vi "STATUS_API.vi"(0 "modpath":path, 7 "Cmd":string, 11 "error in":errorcluster) -> (4 "ImmedReplyString":string, 15 "error out":errorcluster)   [LabVIEW 2016]
uses:
  DBSHAND/private/vis/DatabaseHand_Element_Set(string).vi
  DBSHAND/private/vis/DatabaseHand_Element_Set(bool).vi
panel:
  in  "Status server name":string="STATUS_Main.vi"
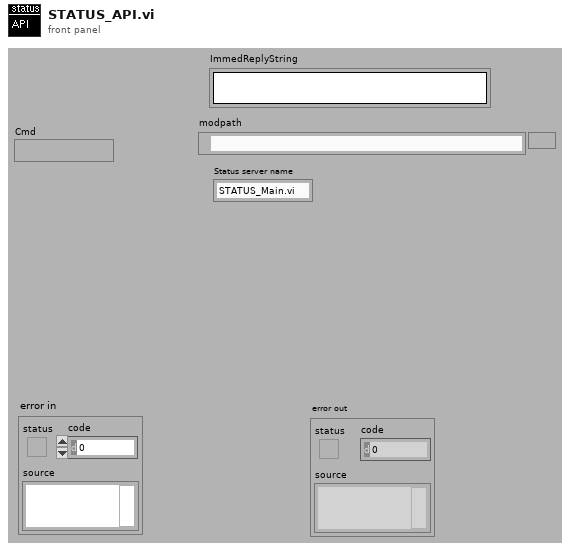
[diagram p1: front panel]
types:
  T1 = typedef "DatabaseHand_RefNum.ctl" = refnum<vi>
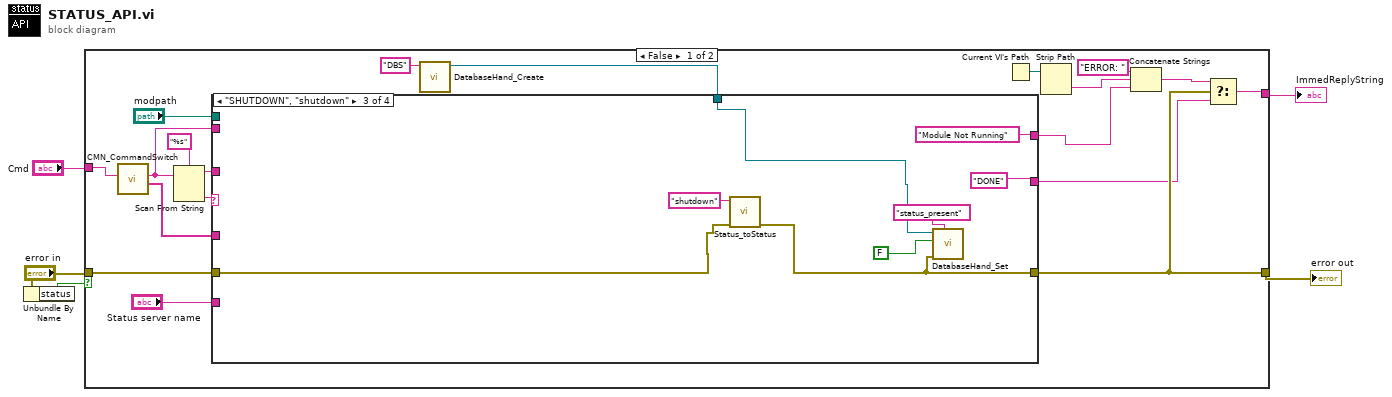
[diagram p0: block diagram]
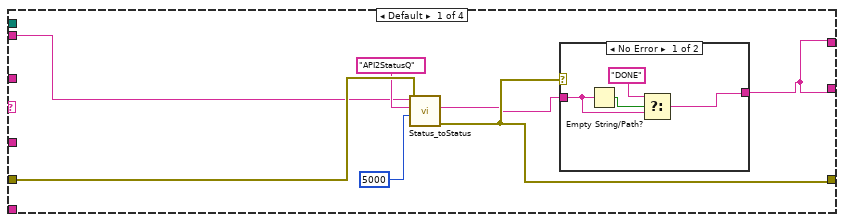
[diagram p2: hidden frame]
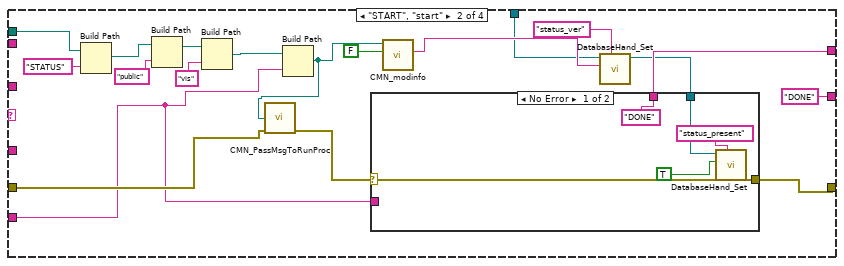
[diagram p4: hidden frame]
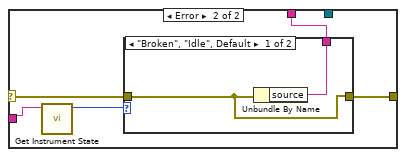
[diagram p5: hidden frame]
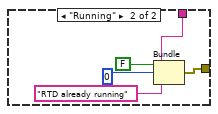
[diagram p6: hidden frame]
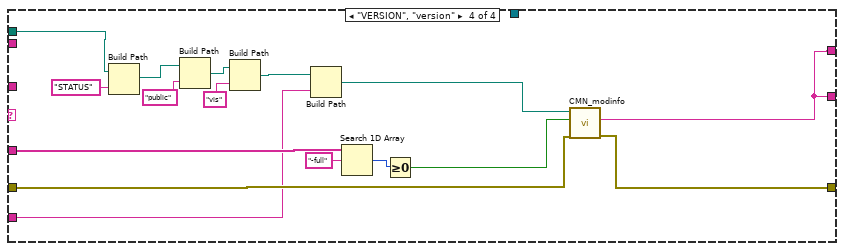
[diagram p7: hidden frame]
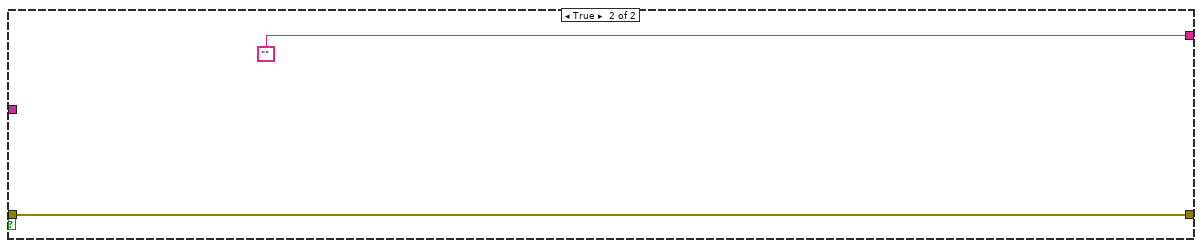
[diagram p8: hidden frame]
diagram:
  n1 = Unbundle By Name("error in") -> ("status"=w3:bool)
  n2 = case shown="False" w3 {
    tunnel: "error in" -> [w24 w97]
    tunnel: [w17 w97] -> w1
    tunnel: [w16 ""] -> w5
    tunnel: "Cmd" -> [w13 _]
    frame False {
      n3 = call "CMN_CommandSwitch.vi"("command in"=w13) -> ("swhitches"=w12:string[], "command out"=w6:string)  [unwired: 1 in, 8 out]
      n4 = Scan From String(format string="%s" ("Format String"), input string=w6) -> (remaining string=w11:string, output 1=w23:string)  [unwired: 2 in, 3 out]
      n5 = call "DatabaseHand_Create.vi"("Name"="DBS") -> ("Database RefNum out"=w9:T1)  [unwired: 1 in, 9 out]
      n6 = case shown="\"SHUTDOWN\", \"shutdown\"" w23 {
        tunnel: w24 -> [w31 w41 w72 w91]
        tunnel: [w30 w54 w73 w90] -> w17
        tunnel: [w28 w47 "Module Not Running" w89] -> w15
        tunnel: [w28 "DONE" "DONE" w89] -> w14
        tunnel: w12 -> [_ _ _ w92]
        tunnel: w11 -> [_ _ _ _]
        tunnel: w9 -> [_ w40 w74 _]
        tunnel: "modpath" -> [_ w38 _ w84]
        tunnel: "Status server name" -> [_ w37 _ w80]
        tunnel: w6 -> [w25 _ _ _]
        frame Default {
          n7 = call "Status_toStatus.vi"("error in (no error)"=w31, "ms timeout (-1)"=5000, "responseQ"="API2StatusQ", "Command"=w25) -> ("error out"=w30:errorcluster, "response"=w29:string)  [unwired: 6 out]
          n8 = case shown="No Error" w30 {
            tunnel: w29 -> [w32 w36]
            tunnel: [w33 w36] -> w28
            frame No Error {
              n9 = Empty String/Path?(string/path=w32) -> (empty?=w35:bool)
              n10 = Select(t="DONE", s=w35, f=w32) -> (s? t:f=w33:string)
            }
            frame Error {
            }
          }
        }
        frame "START", "start" {
          n11 = Build Path(base path=w38, name or relative path="STATUS") -> (appended path=w51:path)
          n12 = Build Path(base path=w51, name or relative path="public") -> (appended path=w49:path)
          n13 = Build Path(base path=w49, name or relative path="vis") -> (appended path=w43:path)
          n14 = Build Path(base path=w43, name or relative path=w37) -> (appended path=w42:path)
          n15 = call "CMN_PassMsgToRunProc.vi"("VItoRun"=w42, "error in (no error)"=w41) -> ("error out"=w55:errorcluster)  [unwired: 1 in, 12 out]
          n16 = call "CMN_modinfo.vi"("full"=FALSE, "caller path"=w42) -> ("INFO"=w45:string)  [unwired: 1 in, 8 out]
          n17 = call-poly "DatabaseHand_Set.vi"("name"="status_ver", "value"=w45, "Database RefNum in"=w40) -> ("Database RefNum out"=w39:T1)  [unwired: 5 in, 3 out]
          n18 = case shown="No Error" w55 {
            selector: w55 -> [w59 w65]
            tunnel: [w59 w62] -> w54
            tunnel: ["DONE" ("source") w64] -> w47
            tunnel: w37 -> [_ w61]
            tunnel: w39 -> [w56 _]
            frame No Error {
              n19 = call-poly "DatabaseHand_Set.vi"("name"="status_present", "value"=TRUE ("full"), "Database RefNum in"=w56) -> ()  [unwired: 5 in, 4 out]
            }
            frame Error {
              n20 = call <vilib>:"Get Instrument State.vi"("VI name"=w61) -> ("vi state"=w63:enum32{"Broken", "Idle", "Running"})  [unwired: 1 in, 9 out]
              n21 = case shown="\"Broken\", \"Idle\", Default" w63 {
                tunnel: w65 -> [w66 _]
                tunnel: [w67 w68] -> w64
                tunnel: [w66 w71] -> w62
                frame "Broken", "Idle", Default {
                  n22 = Unbundle By Name(w66) -> ("source"=w67:string)
                }
                frame "Running" {
                  w68 = "RTD already running"
                  n23 = Bundle(FALSE, 0, w68) -> (w71:errorcluster)  [unwired: 1 out]
                }
              }
            }
          }
        }
        frame "SHUTDOWN", "shutdown" {
          n24 = call "Status_toStatus.vi"("error in (no error)"=w72, "Command"="shutdown") -> ("error out"=w73:errorcluster)  [unwired: 3 in, 6 out]
          n25 = call-poly "DatabaseHand_Set.vi"("name"="status_present", "error in (no error)"=w73, "value"=FALSE ("full"), "Database RefNum in"=w74) -> ()  [unwired: 4 in, 4 out]
        }
        frame "VERSION", "version" {
          n26 = Build Path(base path=w84, name or relative path="STATUS") -> (appended path=w82:path)
          n27 = Build Path(base path=w82, name or relative path="public") -> (appended path=w81:path)
          n28 = Build Path(base path=w81, name or relative path="vis") -> (appended path=w85:path)
          n29 = Build Path(base path=w85, name or relative path=w80) -> (appended path=w83:path)
          n30 = Search 1D Array(1D array=w92, element="-full") -> (index of element=w94:i32)  [unwired: 1 out]
          n31 = Greater Or Equal To 0?(x=w94) -> (x >= 0?=w93:bool)
          n32 = call "CMN_modinfo.vi"("error in (no error)"=w91, "full"=w93, "caller path"=w83) -> ("error out"=w90:errorcluster, "INFO"=w89:string)  [unwired: 7 out]
        }
      }
      n33 = Current VI's Path() -> (path=w20:path)
      n34 = Strip Path(path=w20) -> (name=w19:string)  [unwired: 1 out]
      n35 = Concatenate Strings("ERROR: ", w19, w15) -> (w18:string)
      n36 = Select(t=w18, s=w17, f=w14) -> (s? t:f=w16:string)
    }
    frame True {
    }
  }
  "error out" <- w1
  "ImmedReplyString" <- w5
